vi "FSMGoTo.vi"(1 "Target Value (V)":dbl format="%0.2f", 2 "FSM Task":refnum<k21>) -> (0 "error out":errorcluster)   [LabVIEW 2019]
uses:
  <vilib>/DAQmx/write.llb/DAQmx Write (Analog DBL 1Chan 1Samp).vi
  <vilib>/DAQmx/miscellaneous.llb/DAQmx Fill In Error Info.vi
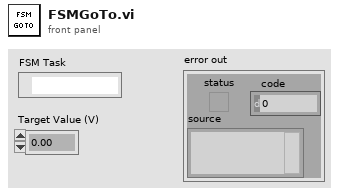
[diagram p1: front panel]
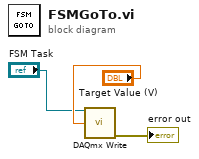
[diagram p0: block diagram]
diagram:
  n1 = call-poly <vilib>:"DAQmx Write.vi"("task/channels in"="FSM Task", "data"="Target Value (V)") -> ("error out"=→"error out":errorcluster)  [unwired: 11 in, 2 out]
